vi "MCCOpen.vi"(9 "Open":bool, 10 "Hardware Settings":T1={"Galvo Channels"="Dev1/ao0:1", "Detector Channels"="Dev1/ai0:2", "Galvo Trigger"="/Dev1/ai/StartTrigger", "Shutter Lines"=["Dev1/port0/line7"], "Max Acquisition Rate"=5000000.0, "Recommended Acquisition Rate"=5000000.0, "Galvo Write Rate"=2500000.0, "Max Timebase Frequency (Hz)"=20000000.0, "MCC Shutter Lines"=[], "Detector Task"="", "Shutter Tasks"=[], "Galvo Task"="", "Digital Image Multiplier"=[100.0, 100.0, -100.0]} {"Max Acquisition Rate" min=0.0 max=5000000.0 step=100000.0}, 11 "index":i32) -> (0 "error out":errorcluster)   [LabVIEW 2012]
uses:
  typedefs/HWsettings.ctl
  <vilib>/ULx/Create Channel.llb/ULx Create Channel (DO-Digital Output).vi
  <vilib>/ULx/Write.llb/ULx Write (Digital Bool 1Line 1Point).vi
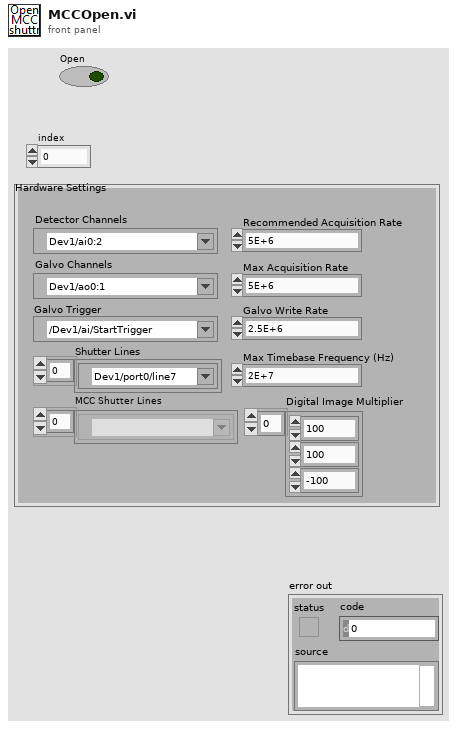
[diagram p1: front panel]
types:
  T1 = typedef "HWsettings.ctl" = cluster{"Galvo Channels":tag, "Detector Channels":tag, "Galvo Trigger":tag, "Shutter Lines":tag[], "Max Acquisition Rate":dbl, "Recommended Acquisition Rate":dbl, "Galvo Write Rate":dbl, "Max Timebase Frequency (Hz)":dbl, "MCC Shutter Lines":refnum<k21>[], "Detector Task":refnum<k21>, "Shutter Tasks":refnum<k21>[], "Galvo Task":refnum<k21>, "Digital Image Multiplier":dbl[]}
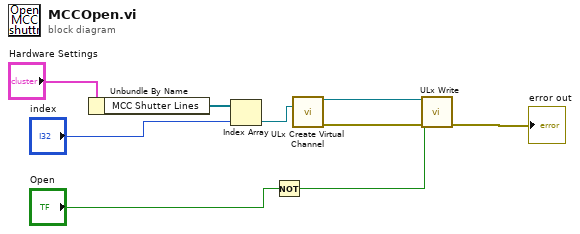
[diagram p0: block diagram]
diagram:
  n1 = Unbundle By Name("Hardware Settings") -> ("MCC Shutter Lines"=w7:refnum<k21>[])
  n2 = Index Array(array=w7, index="index") -> (element=w8:refnum<k21>)
  n3 = Not(x="Open") -> (.not. x?=w3:bool)
  n4 = call-poly <vilib>:"ULx Create Virtual Channel.vi"("lines"=w8) -> ("task out"=w6:refnum<k24>, "error out"=w2:errorcluster)  [unwired: 13 in]
  n5 = call-poly <vilib>:"ULx Write.vi"("task in"=w6, "data"=w3, "error in"=w2) -> ("error out"=→"error out":errorcluster)  [unwired: 10 in, 2 out]
